vi "defender_normal.vi"(9 "balls":T1[](array[typedef]), 10 "IA State":T2={"our_robots"=[], "enemy_robots"=[], "balls"=[], "geometry"={"line_width"=0, "field_length"=0, "field_width"=0, "boundary_width"=0, "referee_width"=0, "goal_width"=0, "goal_depth"=0, "goal_wall_width"=0, "center_circle_radius"=0, "defense_radius"=0, "defense_stretch"=0, "free_kick_from_defense_dist"=0, "penalty_spot_from_field_line_dist"=0, "penalty_line_from_spot_dist"=0}, "IA Judge"={"stage"="", "command"="", "our_goalie_id"=0.0, "enemy_goalie_id"=0.0, "command enum"=enum."Halt", "Time"=enum."Azul"}, "Received Timestamp"=timestamp(0 s since 1904-01-01), "Events"={"Touch"=FALSE, "Ball out"=FALSE, "id touch"=0.0, "Ball out of \nVision"=FALSE, "Ball inside \nGoalie area"=FALSE, "Robot not responding"=FALSE, "Robots responding status"=[1.0, 1.0, 1.0, 1.0, 1.0, 1.0], "Enemy Ball \nPossession"=FALSE, "Pass State"=FALSE, "id end of pass"=0.0, "Kick"=FALSE, "Id ini Possession"=0.0, "Ball Possesion"=FALSE, "Id Possesion"=0.0, "Direct Kick"=FALSE, "2nd Strk Ativo"=FALSE}}, 11 "Robot in":T3={"id"=0, "function"=enum."Attacker", "x"=0.0, "y"=0.0, "orientation"=0.0, "v_tangent"=0.0, "v_normal"=0.0, "v_ang"=0.0, "kick_x"=0.0, "kick_z"=0.0, "dribble"=FALSE, "Timestamp"=timestamp(0 s since 1904-01-01), "estimatives"={"est_v_tangent"=0.0, "est_v_normal"=0.0, "est_vx"=0.0, "est_vy"=0.0, "Pos Robot Est"=[]}, "dest_x_kick"=0.0, "dest_y_kick"=0.0, "Gap Coord"=[], "States"=enum."Pass", "Path "=[], "Path  Smooth"=[], "Dest"=[]}) -> (3 "Robot out":T3={"id"=0, "function"=enum."Attacker", "x"=0.0, "y"=0.0, "orientation"=0.0, "v_tangent"=0.0, "v_normal"=0.0, "v_ang"=0.0, "kick_x"=0.0, "kick_z"=0.0, "dribble"=FALSE, "Timestamp"=timestamp(0 s since 1904-01-01), "estimatives"={"est_v_tangent"=0.0, "est_v_normal"=0.0, "est_vx"=0.0, "est_vy"=0.0, "Pos Robot Est"=[]}, "dest_x_kick"=0.0, "dest_y_kick"=0.0, "Gap Coord"=[], "States"=enum."Pass", "Path "=[], "Path  Smooth"=[], "Dest"=[]})   [LabVIEW 2018]
uses:
  Core/AI Robot.ctl
  Intel/Functions Enum.ctl
  RoboIME/VSS git/VSS/Intel/AttackerStates.ctl
  Path Planning/RRT/PathDests.ctl
  Path Planning/RRT/PathDest.ctl
  Core/AI Input.ctl
  Core/AI Ball.ctl
  Core/Field Size.ctl
  Core/AI Judge.ctl
  Intel/Command Enum.ctl
  Util/Events/Events.ctl
  <vilib>/Analysis/_algsub.llb/Real Vector Norm.vi
  <vilib>/Analysis/NI_AALPro.lvlib
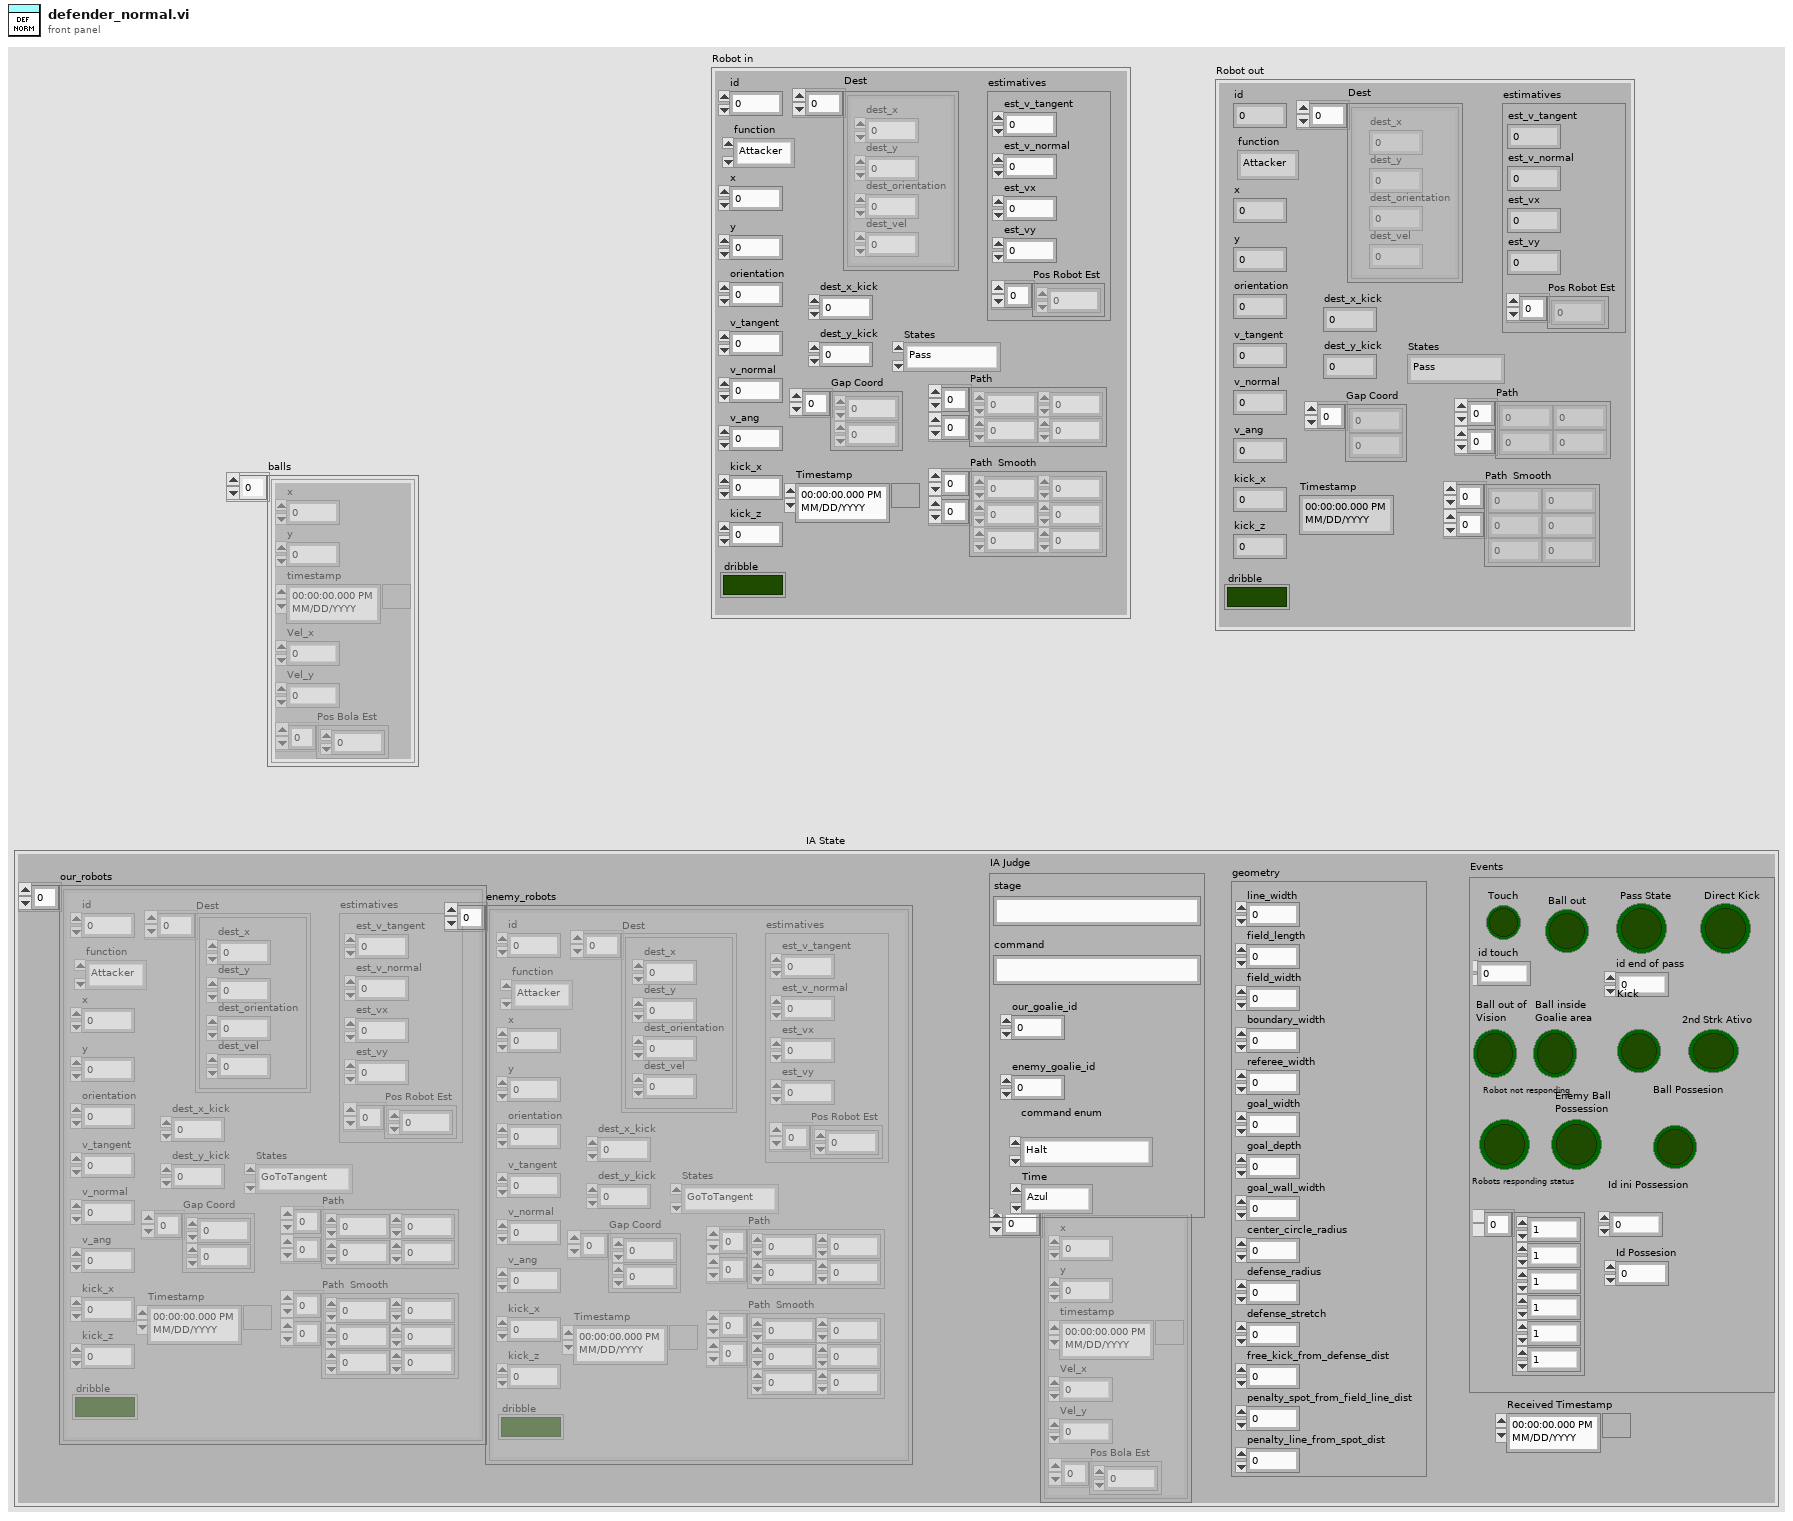
[diagram p1: front panel]
types:
  T1 = typedef "AI Ball.ctl" = cluster{"x":dbl, "y":dbl, "timestamp":timestamp, "Vel_x":dbl, "Vel_y":dbl, "Pos Bola Est":dbl[]}
  T2 = typedef "AI Input.ctl" = cluster{"our_robots":T3[], "enemy_robots":T3[], "balls":T1[], "geometry":T8, "IA Judge":T9, "Received Timestamp":timestamp, "Events":T11}
  T3 = typedef "AI Robot.ctl" = cluster{"id":u32, "function":T4, "x":dbl, "y":dbl, "orientation":dbl, "v_tangent":dbl, "v_normal":dbl, "v_ang":dbl, "kick_x":dbl, "kick_z":dbl, "dribble":bool, "Timestamp":timestamp, "estimatives":cluster{"est_v_tangent":dbl, "est_v_normal":dbl, "est_vx":dbl, "est_vy":dbl, "Pos Robot Est":dbl[]}, "dest_x_kick":dbl, "dest_y_kick":dbl, "Gap Coord":dbl[], "States":T5, "Path ":dbl[][], "Path  Smooth":dbl[][], "Dest":T6}
  T4 = typedef "Functions Enum.ctl" = enum16{"2nd Striker", "Attacker", "Goalie", "Defender", "Striker", "Goto 0", "Dummy", "Kicker", "ZigZag 0", "ZigZag 1", "ZigZag 2", "ZigZag 3", "ZigZag 4", "ZigZag 5", "ZigZag 6", "ZigZag 7", "ZigZag 8", ""}
  T5 = typedef "AttackerStates.ctl" = enum16{"Pass", "GoToTangent", "BallGetting", "GoToKick", "Rotate anti-clockwise", "Rotate Clockwise", ""}
  T6 = typedef "PathDests.ctl" = T7[]
  T7 = typedef "PathDest.ctl" = cluster{"dest_x":dbl, "dest_y":dbl, "dest_orientation":dbl, "dest_vel":dbl}
  T8 = typedef "Field Size.ctl" = cluster{"line_width":u32, "field_length":u32, "field_width":u32, "boundary_width":u32, "referee_width":u32, "goal_width":u32, "goal_depth":u32, "goal_wall_width":u32, "center_circle_radius":u32, "defense_radius":u32, "defense_stretch":u32, "free_kick_from_defense_dist":u32, "penalty_spot_from_field_line_dist":u32, "penalty_line_from_spot_dist":u32}
  T9 = typedef "AI Judge.ctl" = cluster{"stage":string, "command":string, "our_goalie_id":dbl, "enemy_goalie_id":dbl, "command enum":T10, "Time":enum16{"Azul", "Amarelo"}}
  T10 = typedef "Command Enum.ctl" = enum16{"Halt", "Stop", "Force Start", "PKA Normal Start", "Prepare Kickoff Ally", "PKE Normal Start", "Prepare Kickoff Enemy", "Prepare Penalty Ally", "PPA Normal Start", "Prepare Penalty Enemy", "PPE Normal Start", "Direct Free Enemy", "Direct Free Ally", "Indirect Free Enemy", "Indirect Free Ally", "Timeout Enemy", "Timeout Ally", "Goal Enemy", "Goal Ally", "Ball Placement Enemy", "Ball Placement Ally", "Normal Half Time", "Extra Time Break", "Extra Half Time", "None", "Post Game"}
  T11 = typedef "Events.ctl" = cluster{"Touch":bool, "Ball out":bool, "id touch":dbl, "Ball out of \nVision":bool, "Ball inside \nGoalie area":bool, "Robot not responding":bool, "Robots responding status":dbl[], "Enemy Ball \nPossession":bool, "Pass State":bool, "id end of pass":dbl, "Kick":bool, "Id ini Possession":dbl, "Ball Possesion":bool, "Id Possesion":dbl, "Direct Kick":bool, "2nd Strk Ativo":bool}
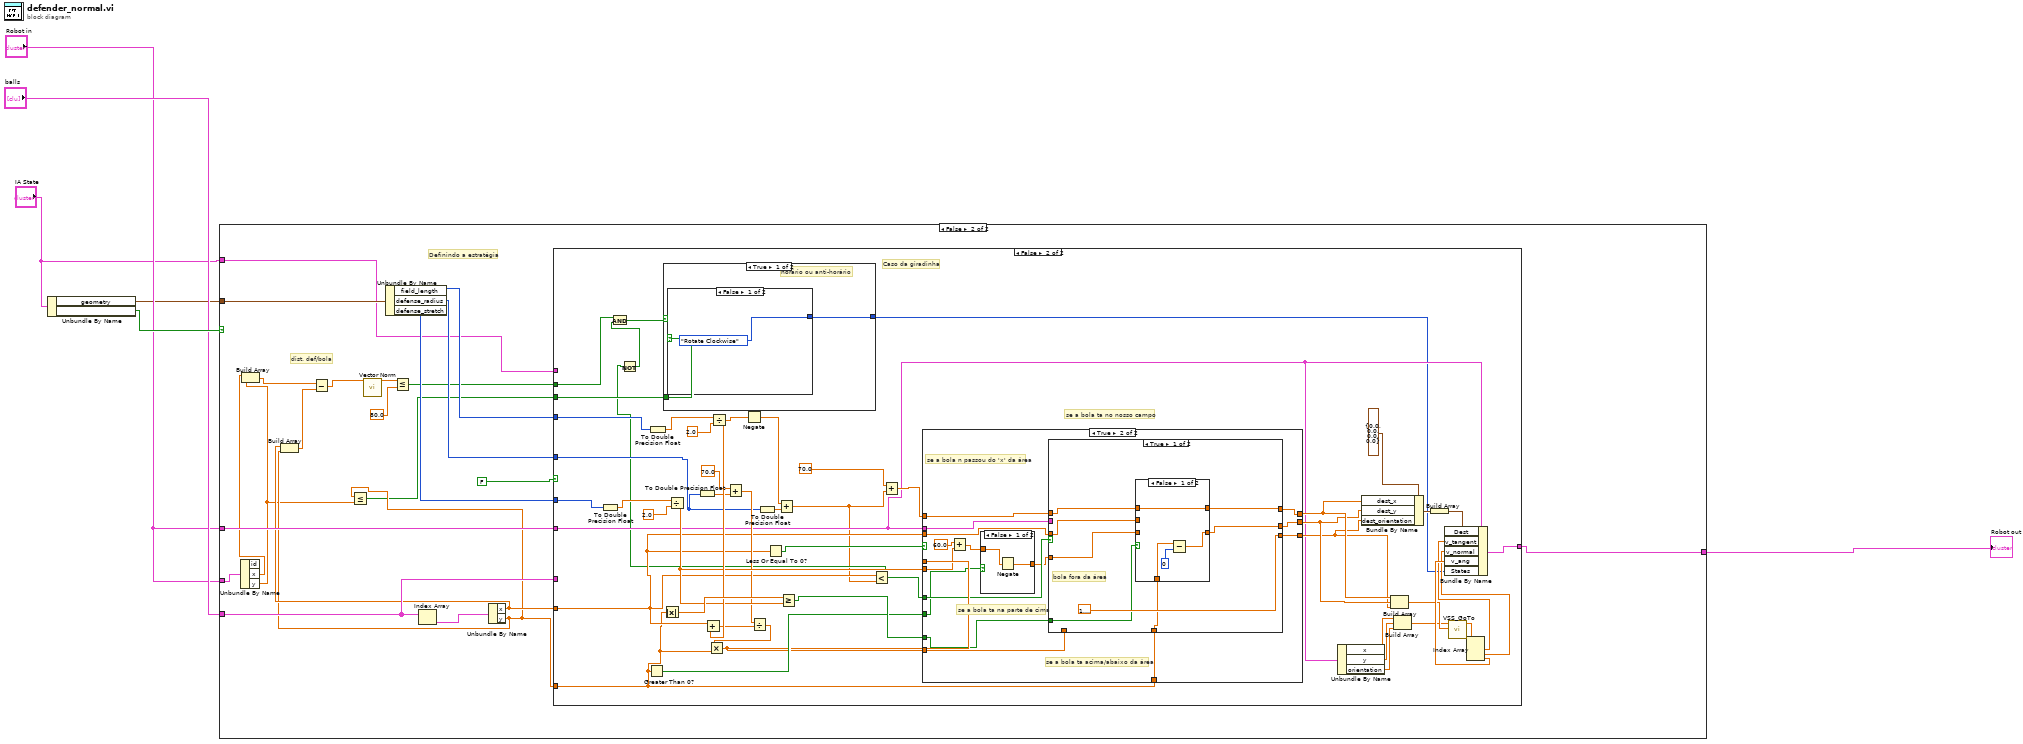
[diagram p0: block diagram]
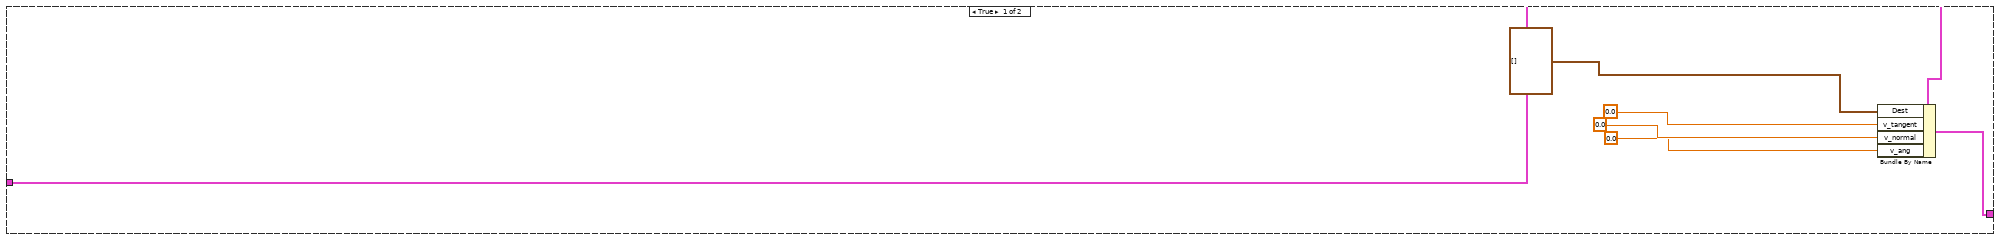
[diagram p2: hidden frame]
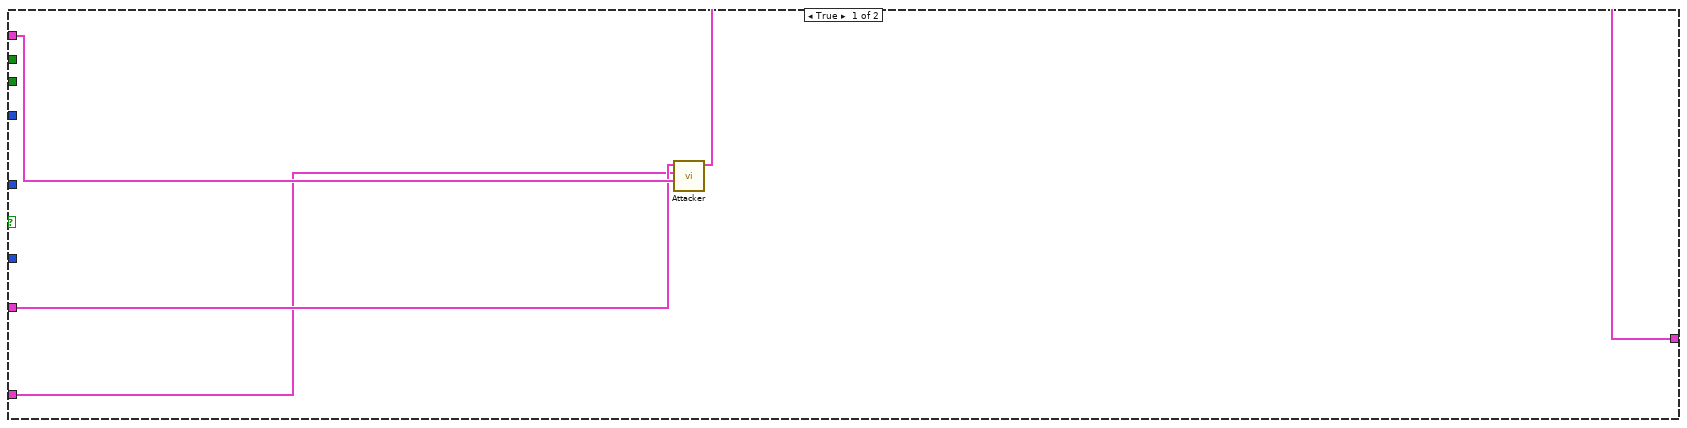
[diagram p3: hidden frame]
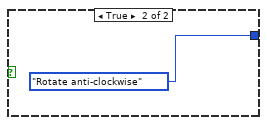
[diagram p4: hidden frame]
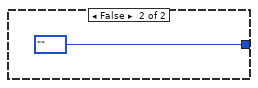
[diagram p5: hidden frame]
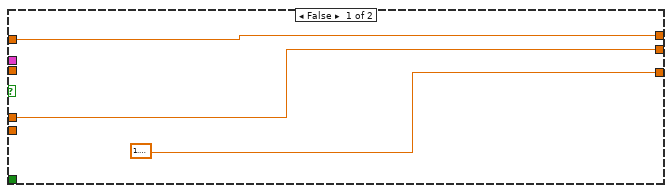
[diagram p6: hidden frame]
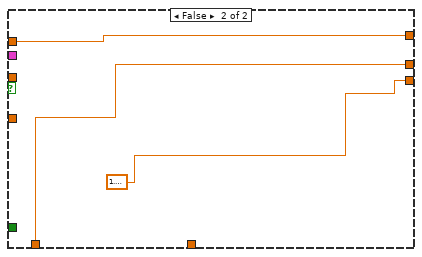
[diagram p9: hidden frame]
diagram:
  n1 = Unbundle By Name("IA State") -> ("geometry"=w3:T8, "Events.Ball out of \nVision"=w6:bool)
  n2 = case shown="False" w6 {
    tunnel: "Robot in" -> [w11 w34]
    tunnel: "balls" -> [_ w26]
    tunnel: "Robot in" -> [_ w32]
    tunnel: w3 -> [_ w31]
    tunnel: "IA State" -> [_ w27]
    tunnel: [w12 w25] -> w1
    frame True {
      n3 = Bundle By Name(cluster=w11, "Dest"=T7[] [], "v_tangent"=0.0, "v_normal"=0.0, "v_ang"=0.0) -> (w12:T3)
    }
    frame False {
      # "dist. def/bola"
      # "Definindo a estratégia"
      n4 = Unbundle By Name(w32) -> ("x"=w22:dbl, "y"=w14:dbl)  [unwired: 1 out]
      n5 = Build Array(w22, w14) -> (w21:dbl[])
      n6 = Unbundle By Name(w31) -> ("field_length"=w30:u32, "defense_radius"=w29:u32, "defense_stretch"=w28:u32)
      n7 = Index Array(array=w26) -> (element=w33:T1)  [unwired: 1 in]
      n8 = Unbundle By Name(w33) -> ("x"=w23:dbl, "y"=w15:dbl)
      n9 = Build Array(w23, w15) -> (w20:dbl[])
      n10 = Subtract(x=w21, y=w20) -> (x-y=w19:dbl[])
      n11 = Less Or Equal?(x=w15, y=w14) -> (x <= y?=w13:bool)
      n12 = call-poly <vilib>:"Vector Norm.vi"("Input Vector"=w19) -> ("norm"=w18:dbl)  [unwired: 9 in, 1 out]
      n13 = Less Or Equal?(x=w18, y=80.0) -> (x <= y?=w16:bool)
      n14 = case shown="False" FALSE {
        tunnel: w34 -> [w37 w54]
        tunnel: w23 -> [_ w71]
        tunnel: w15 -> [_ w70]
        tunnel: w30 -> [_ w52]
        tunnel: w29 -> [_ w49]
        tunnel: w28 -> [_ w46]
        tunnel: w27 -> [w38 _]
        tunnel: w26 -> [w35 _]
        tunnel: [w36 w53] -> w25
        tunnel: w16 -> [_ w44]
        tunnel: w13 -> [_ w42]
        frame True {
          n15 = call "Attacker.vi"("IA State"=w38, "balls"=w35, "Robot in"=w37) -> ("Robot out"=w36:T3)  [unwired: 8 in]
        }
        frame False {
          # "Caso da giradinha"
          # "se a bola ta no nosso campo"
          n16 = To Double Precision Float(number=w46) -> (double precision float=w45:dbl)
          n17 = Greater Than 0?(x=w70) -> (x > 0?=w80:bool)
          n18 = To Double Precision Float(number=w52) -> (double precision float=w51:dbl)
          n19 = Absolute Value(x=w70) -> (abs(x)=w86:dbl)
          n20 = Divide(x=w45, y=2.0) -> (x/y=w76:dbl)
          n21 = To Double Precision Float(number=w49) -> (double precision float=w50:dbl)
          n22 = Divide(x=w51, y=2.0) -> (x/y=w78:dbl)
          n23 = Add(x=w71, y=w78) -> (x+y=w77:dbl)
          n24 = Add(x=70.0, y=w50) -> (x+y=w74:dbl)
          n25 = Negate(x=w78) -> (-x=w85:dbl)
          n26 = Divide(x=w74, y=w77) -> (x/y=w83:dbl)
          n27 = Multiply(x=w83, y=w70) -> (x*y=w73:dbl)
          n28 = To Double Precision Float(number=w49) -> (double precision float=w48:dbl)
          n29 = Less Or Equal To 0?(x=w71) -> (x <= 0?=w79:bool)
          n30 = Add(x=w85, y=w48) -> (x+y=w39:dbl)
          n31 = Greater Or Equal?(x=w86, y=w76) -> (x >= y?=w82:bool)
          n32 = Less?(x=w71, y=w39) -> (x < y?=w41:bool)
          n33 = Not(x=w41) -> (.not. x?=w40:bool)
          n34 = Compound Arithmetic op=AND(w44, w40) -> (w43:bool)
          n35 = case shown="True" w43 {
            tunnel: [w88 AttackerStates."" ("States")] -> w47
            tunnel: w42 -> [w89 _]
            frame True {
              # "horário ou anti-horário"
              n36 = case shown="False" w89 {
                tunnel: [AttackerStates."Rotate Clockwise" ("States") AttackerStates."Rotate anti-clockwise" ("States")] -> w88
                frame False {
                }
                frame True {
                }
              }
            }
            frame False {
            }
          }
          n37 = Add(x=70.0, y=w39) -> (x+y=w72:dbl)
          n38 = case shown="True" w79 {
            tunnel: w54 -> [_ w110]
            tunnel: w72 -> [w95 w109]
            tunnel: w41 -> [_ w108]
            tunnel: w80 -> [_ w107]
            tunnel: w76 -> [_ w100]
            tunnel: w71 -> [_ w106]
            tunnel: w73 -> [w94 _]
            tunnel: w82 -> [_ w98]
            tunnel: [w95 w105] -> w57
            tunnel: [w94 w104] -> w56
            tunnel: [1.5707963267948966 w103] -> w55
            tunnel: w70 -> [_ w99]
            tunnel: w73 -> [_ w96]
            frame False {
            }
            frame True {
              # "se a bola ta acima/abaixo da área"
              # "se a bola n passou do 'x' da área"
              # "se a bola ta na parte de cima"
              n39 = Add(x=60.0, y=w100) -> (x+y=w102:dbl)
              n40 = case shown="False" w107 {
                tunnel: w102 -> [w112 w113]
                tunnel: [w111 w113] -> w97
                frame False {
                  n41 = Negate(x=w112) -> (-x=w111:dbl)
                }
                frame True {
                }
              }
              n42 = case shown="True" w108 {
                tunnel: w110 -> [_ _]
                tunnel: w97 -> [w117 _]
                tunnel: w109 -> [w116 w130]
                tunnel: w106 -> [w114 _]
                tunnel: [w115 w130] -> w105
                tunnel: [w120 w128] -> w104
                tunnel: [1.5707963267948966 1.5707963267948966] -> w103
                tunnel: w98 -> [w118 _]
                tunnel: w99 -> [w119 _]
                tunnel: w96 -> [_ w128]
                frame True {
                  # "bola fora da área"
                  n43 = case shown="False" w118 {
                    tunnel: w117 -> [_ w127]
                    tunnel: [w122 w127] -> w120
                    tunnel: w119 -> [w124 _]
                    tunnel: w116 -> [w125 _]
                    tunnel: [w125 w126] -> w115
                    tunnel: w114 -> [_ w126]
                    frame False {
                      n44 = Subtract(x=w124, y=0) -> (x-y=w122:dbl)
                    }
                    frame True {
                    }
                  }
                }
                frame False {
                }
              }
            }
          }
          n45 = Unbundle By Name(w54) -> ("x"=w61:dbl, "y"=w58:dbl, "orientation"=w59:dbl)
          n46 = Bundle By Name(cluster=T7 {"dest_x"=0.0, "dest_y"=0.0, "dest_orientation"=0.0, "dest_vel"=0.0} ("element"), "dest_x"=w57, "dest_y"=w56, "dest_orientation"=w55) -> (w64:T7)
          n47 = Build Array(w57, w56, w55) -> (w62:dbl[])
          n48 = Build Array(w61, w58, w59) -> (w60:dbl[])
          n49 = Build Array(w64) -> (w66:T7[])
          n50 = call "VSS_GoTo.vi"("SetPoint"=w62, "Position"=w60) -> ("Output Vel"=w63:dbl[])  [unwired: 9 in]
          n51 = Index Array(array=w63) -> (element #1=w67:dbl, element #2=w68:dbl, element #3=w69:dbl)  [unwired: 3 in]
          n52 = Bundle By Name(cluster=w54, "Dest"=w66, "v_tangent"=w67, "v_normal"=w68, "v_ang"=w69, "States"=w47) -> (w53:T3)
        }
      }
    }
  }
  "Robot out" <- w1
